vi "FWHM-Fast.vi"() -> ()   [LabVIEW 2014]
doc: "André Romero - 2017\nandretec@ifsc.usp.br"
panel:
  out "FWHM":dbl=7.6633162264068915
  in  "stop":bool
  out "XY Graph":T1(graph)
  out "Length":i32=2048
  in  "Correct Electrical Dark":bool=TRUE
  in  "Integration Time (ms)":i32=100
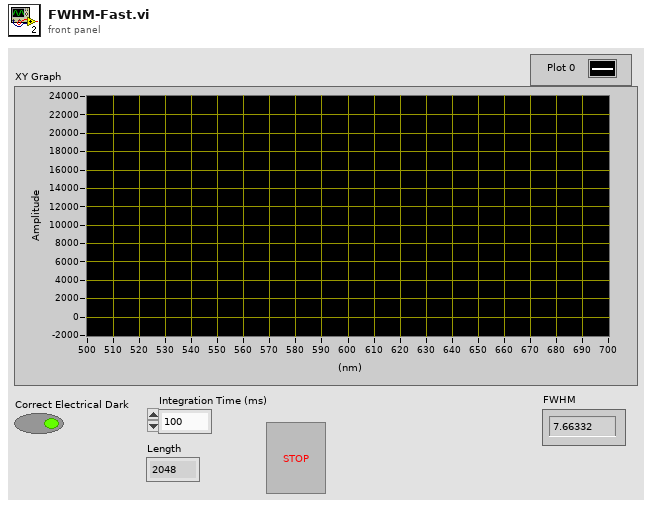
[diagram p1: front panel]
types:
  T1 = cluster{"WL Values":dbl[], "Spectrum Values":dbl[]}
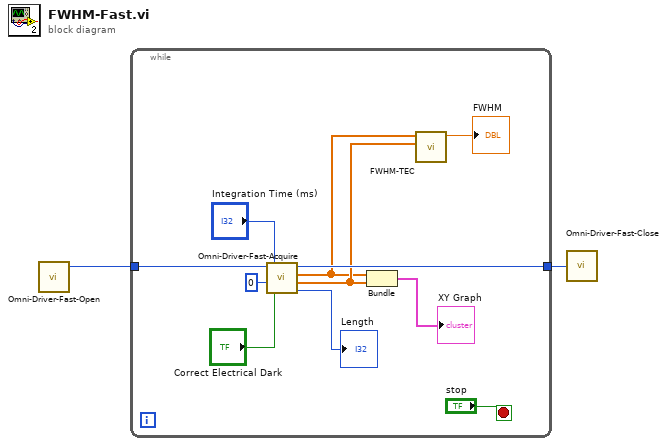
[diagram p0: block diagram]
diagram:
  n1 = call "Omni-Driver-Fast-Open.vi"() -> ("Wrapper Out"=w2:u32)  [unwired: 4 in, 1 out]
  n2 = while {
    tunnel: w2 -> [w13]
    tunnel: [w12] -> w1
    stop <- "stop" stop-if-true
    n3 = call "Omni-Driver-Fast-Acquire.vi"("Correct Electrical Dark"="Correct Electrical Dark", "Spectrometer number"=0, "Integration Time (ms)"="Integration Time (ms)", "Wrapper"=w13) -> ("Length"=→"Length":i32, "Spectrum Values"=w5:dbl[], "WL Values"=w4:dbl[], "Wrapper Out"=w12:u32)
    n4 = Bundle("WL Values"=w4, "Spectrum Values"=w5) -> (→"XY Graph":T1)  [unwired: 1 in]
    n5 = call "FWHM-TEC.vi"("Y values"=w5, "WL values"=w4) -> ("FWHM"=→"FWHM":dbl)  [unwired: 9 in]
  }
  n6 = call "Omni-Driver-Fast-Close.vi"("Wrapper In"=w1) -> ()  [unwired: 1 in]
